vi "字符串转换为数组.vi"(11 "查询内容":string) -> (3 "列首":string[](array[string]))   [LabVIEW 2013]
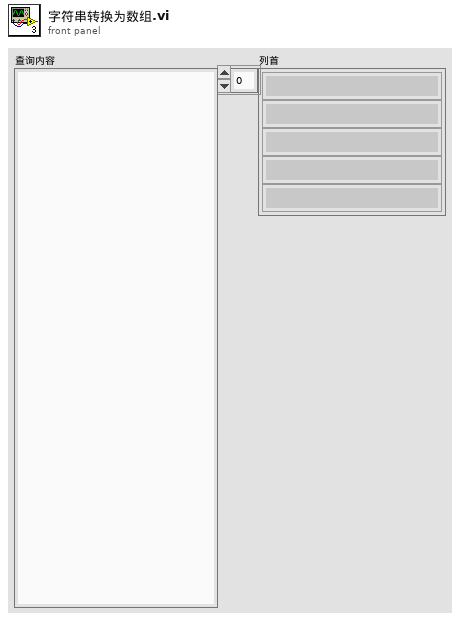
[diagram p1: front panel]
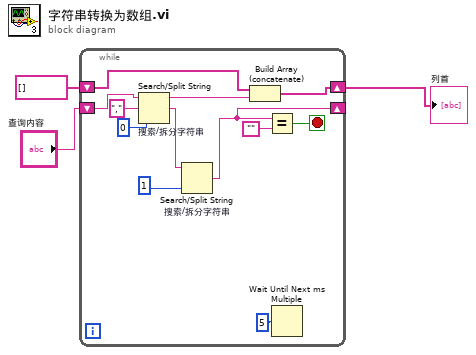
[diagram p0: block diagram]
diagram:
  n1 = while {
    shift-right: [w4] -> _
    shift-left: "查询内容" -> [w14]
    shift-right: [w12] -> w1
    shift-left: string[] [] -> [w13]
    stop <- w9 stop-if-true
    n2 = Search/Split String "搜索/拆分字符串"(string=w14, search string/char (-)="," ("搜索字符串/字符(-)"), offset (0)=0 ("偏移量(0)")) -> (substring before match=w11:string, match + rest of string=w6:string)  [unwired: 1 out]
    n3 = Search/Split String "搜索/拆分字符串"(string=w6, offset (0)=1 ("长度（剩余）")) -> (match + rest of string=w4:string)  [unwired: 1 in, 2 out]
    n4 = Build Array (concatenate)(w13, w11) -> (w12:string[])
    n5 = Equal?(x=w4, y="") -> (x = y?=w9:bool)
    n6 = Wait Until Next ms Multiple(millisecond multiple=u32 5 ("毫秒倍数")) -> ()  [unwired: 1 out]
  }
  "列首" <- w1
